vi "STM Write Message (UDP).vi"(4 "Address":cluster{"address":u32, "port":u16}, 6 "Options":T1={"Ignore Timeout Error"=TRUE, "timeout ms (1000)"=1000}, 8 "error in (no error)":errorcluster, 9 "Data":string, 10 "Name":string, 11 "Connection Info":T2) -> (0 "error out":errorcluster, 3 "Connection Info Out":T2)   [LabVIEW 2010]
doc: "This VI writes a package of data to a remote computer. It prepends a meta data ID number to each packet. \n\nThe data must be passed in as a String. The calling VI is responsible for flattening the desired data to a string before passing it to this VI."
uses:
  stm_UDP Connection Info.ctl
  stm_MetaDataElement.ctl
  stm_UDP Write Options.ctl
  NI STM.lvlib
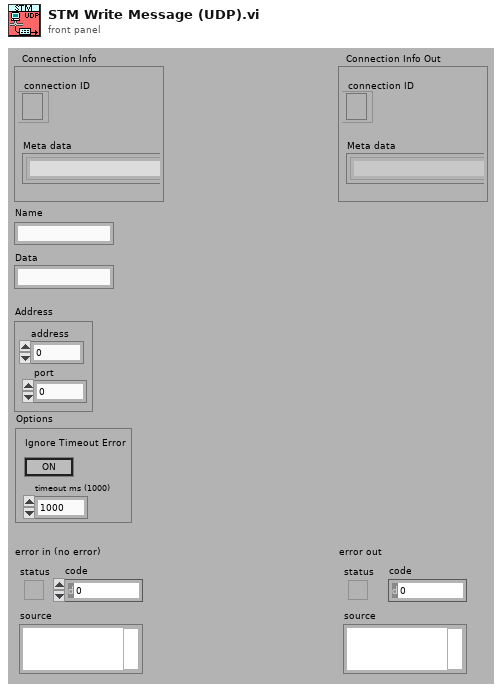
[diagram p1: front panel]
types:
  T1 = typedef "stm_UDP Write Options.ctl" = cluster{"Ignore Timeout Error":bool, "timeout ms (1000)":i32}
  T2 = typedef "stm_UDP Connection Info.ctl" = cluster{"connection ID":refnum<k16>, "Meta data":T3[]}
  T3 = typedef "stm_MetaDataElement.ctl" = string
  T4 = typedef "NI STM.lvlib/UDP Connection Info.ctl" = cluster{"connection ID":refnum<k16>, "Meta data":T5[]}
  T5 = typedef "NI STM.lvlib/MetaDataElement.ctl" = string
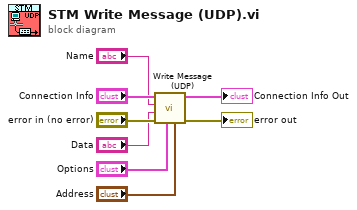
[diagram p0: block diagram]
diagram:
  n1 = call "Write Message (UDP).vi"("Address"="Address", "Options"="Options", "error in"="error in (no error)", "Data"="Data", "Name"="Name", "Connection Info"="Connection Info") -> ("error out"=→"error out":errorcluster, "Connection Info Out"=→"Connection Info Out":T4)  [unwired: 4 in]
